vi "Create Queue.vi"(8 "error in (no error)":errorcluster) -> (0 "error out":errorcluster)   [LabVIEW 2022 SP3]
doc: "Creates the module's command queue. This queue is used to issue commands (or requests) to the module. The queue size is -1 (unlimited).\n\nThis VI raises an error if a queue of the same name already exists. For example, this can happen if the 'Create' VI is called twice in a row, or called twice without 'Destroy' having been called in between.\n\nRecommended use: Call 'Create' only once during the lifetime of the app. Call it as part of the module init routine (before MHL)."
uses:
  Message.ctl
  Command.ctl
panel:
  # "Development\ncontrols/indicators useful for development and testing, but which are not outputs of the VI"
  # "Input\nInputs to the VI"
  # "Output\nOutputs of the VI"
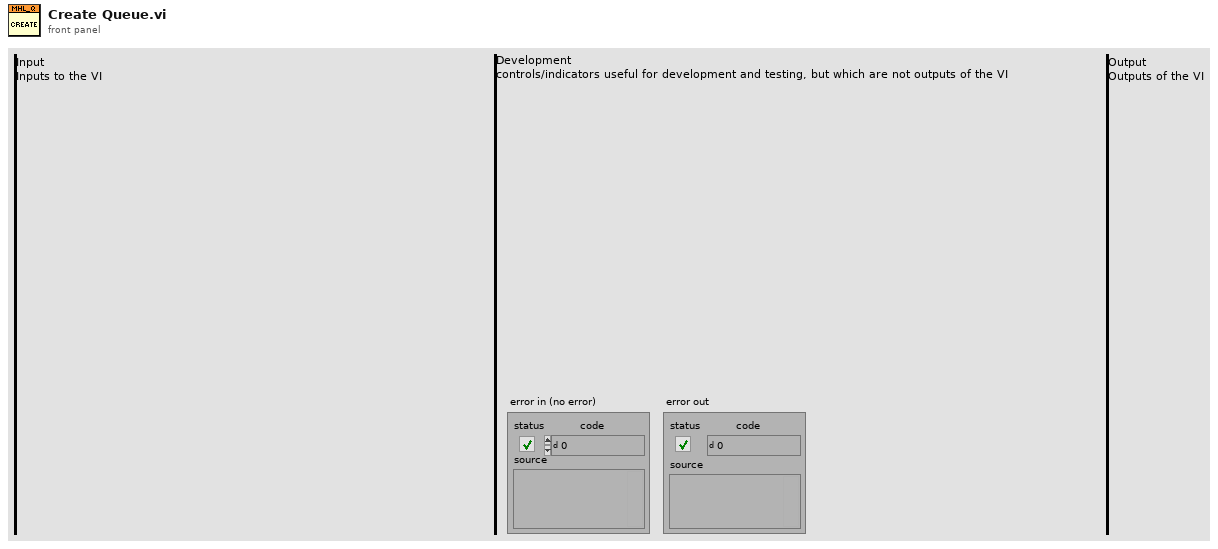
[diagram p1: front panel]
types:
  T1 = typedef "Message.ctl" = cluster{"Command":T2, "Data":variant}
  T2 = typedef "Command.ctl" = enum16{"Init Module", "Close Module", "Local Error Handler", "Command 1 (replace me)", "Command 2 (replace me)", "Command 3 (replace me)"}
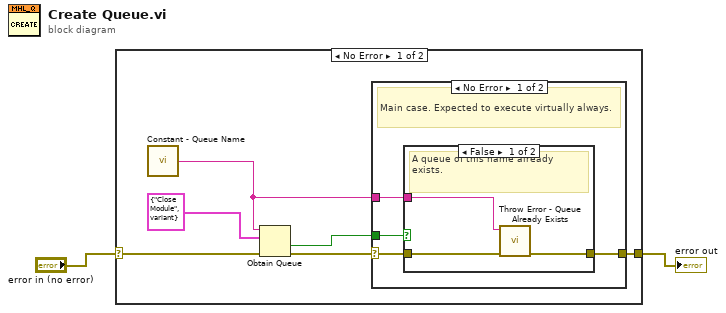
[diagram p0: block diagram]
diagram:
  n1 = case shown="No Error" "error in (no error)" {
    selector: "error in (no error)" -> [w8 w18]
    tunnel: [w5 w18] -> w1
    frame No Error {
      n2 = call "Constant - Queue Name.vi"() -> ("Queue Name"=w3:string)
      n3 = Obtain Queue(name (unnamed)=w3, element data type=T1 {"Command"=enum."Close Module", "Data"=variant} ("Queue Message"), error in (no error)=w8) -> (created new?=w4:bool, error out=w6:errorcluster)  [unwired: 2 in, 1 out]
      n4 = case shown="No Error" w6 {
        selector: w6 -> [w12 w17]
        tunnel: [w11 w17] -> w5
        tunnel: w4 -> [w10 _]
        tunnel: w3 -> [w9 _]
        frame No Error {
          # "Main case. Expected to execute virtually always."
          n5 = case shown="False" w10 {
            tunnel: w12 -> [w15 w16]
            tunnel: [w14 w16] -> w11
            tunnel: w9 -> [w13 _]
            frame False {
              # "A queue of this name already exists."
              n6 = call "Throw Error - Queue Already Exists.vi"("error in (no error)"=w15, "Queue Name"=w13) -> ("error out"=w14:errorcluster)  [unwired: 9 in]
            }
            frame True {
              # "Do nothing."
              # "A new queue was created. This is expected. Main case."
            }
          }
        }
        frame Error {
          # "Pass the error unaltered."
          # "Error upstream."
        }
      }
    }
    frame Error {
    }
  }
  "error out" <- w1
